vi "defineMove.vi"(0 "Lista_mão":dbl[][](array[numeric]), 3 "Lista_ponta":dbl[](array[numeric])) -> (6 "Idx mão":i32, 7 "Idx ponta":i32, 10 "Dobrão":bool)   [LabVIEW 2016]
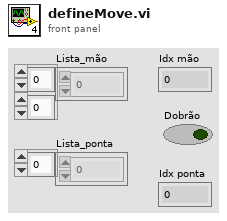
[diagram p1: front panel]
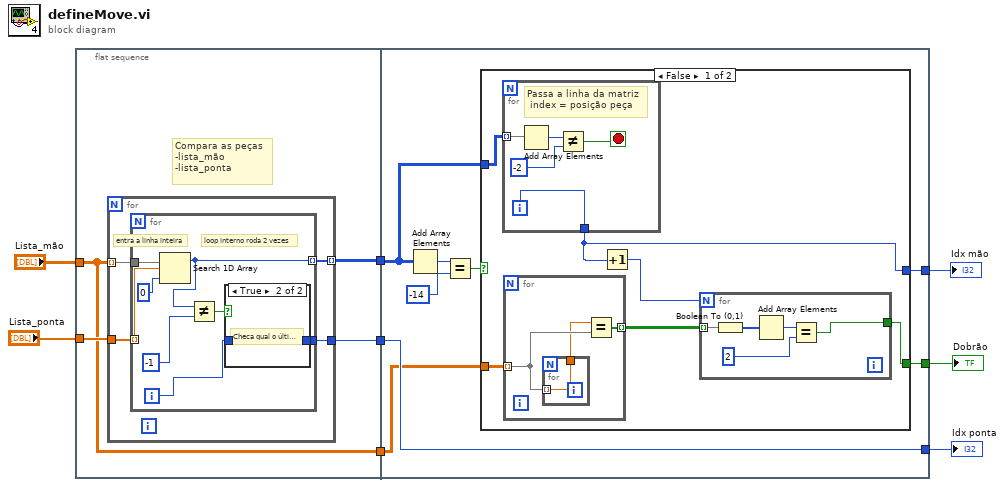
[diagram p0: block diagram]
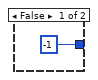
[diagram p2: hidden frame]
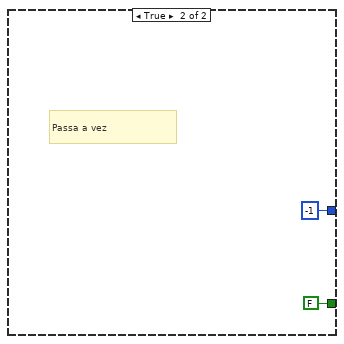
[diagram p3: hidden frame]
diagram:
  n1 = flat-sequence {
    tunnel: "Lista_mão" -> [w9]
    tunnel: "Lista_ponta" -> [w12]
    tunnel: [w11] -> w8
    tunnel: [w10] -> w7
    tunnel: [w9] -> w6
    tunnel: w8 -> [w31]
    tunnel: [w30] -> w4
    tunnel: [w29] -> w3
    tunnel: w7 -> [w28]
    tunnel: [w28] -> w5
    tunnel: w6 -> [w27]
    frame #0 {
      # "Compara as peças\n-lista_mão\n-lista_ponta"
      n2 = for {
        tunnel: w9 -> [w16] mode=indexing
        tunnel: w12 -> [w15]
        tunnel: [w14] -> w11 mode=indexing
        tunnel: [w13] -> w10
        # "entra a linha inteira"
        n3 = for {
          tunnel: w16 -> [w24]
          tunnel: w15 -> [w23] mode=indexing
          tunnel: [w20] -> w14 mode=indexing
          tunnel: [w18] -> w13
          i -> [w17]
          # "loop interno roda 2 vezes"
          n4 = Search 1D Array(1D array=w24, element=w23, start index (0)=0) -> (index of element=w20:i32)
          n5 = Not Equal?(x=w20, y=-1) -> (x != y?=w21:bool)
          n6 = case shown="True" w21 {
            tunnel: w17 -> [_ w26]
            tunnel: [-1 w26] -> w18
            frame False {
            }
            frame True {
              # "Checa qual o último numero da lista mão  \nque é diferente  de -1 e retorna o index da \nlista ponta que deve colocar a peça pegada"
            }
          }
        }
      }
    }
    frame #1 {
      n7 = Add Array Elements(numeric array=w31) -> (sum=w34:i32)
      n8 = Equal?(x=w34, y=-14) -> (x = y?=w32:bool)
      n9 = case shown="False" w32 {
        tunnel: w31 -> [w37 _]
        tunnel: [w36 -1] -> w30
        tunnel: [w38 FALSE] -> w29
        tunnel: w27 -> [w35 _]
        frame False {
          n10 = for {
            tunnel: w37 -> [w54] mode=indexing
            tunnel: [w50] -> w36
            i -> [w50]
            stop <- w52 stop-if-true
            # "Passa a linha da matriz\n index = posição peça"
            n11 = Add Array Elements(numeric array=w54) -> (sum=w53:i32)
            n12 = Not Equal?(x=w53, y=-2) -> (x != y?=w52:bool)
          }
          n13 = for {
            tunnel: w35 -> [w48] mode=indexing
            tunnel: [w46] -> w40 mode=indexing
            n14 = for {
              tunnel: w48 -> [w49] mode=indexing
              tunnel: [w49] -> w47
            }
            n15 = Equal?(x=w47, y=w48) -> (x = y?=w46:bool[])
          }
          n16 = Increment(x=w36) -> (x+1=w39:i32)
          n17 = for {
            N: w39 -> [_]
            tunnel: w40 -> [w45] mode=indexing
            tunnel: [w41] -> w38
            n18 = Boolean To (0,1)(Boolean=w45) -> (0, 1=w44:i16[])
            n19 = Add Array Elements(numeric array=w44) -> (sum=w43:i16)
            n20 = Equal?(x=w43, y=i16 2) -> (x = y?=w41:bool)
          }
        }
        frame True {
          # "Passa a vez"
        }
      }
    }
  }
  "Idx ponta" <- w5
  "Idx mão" <- w4
  "Dobrão" <- w3
